vi "Process data - Overview v2.vi"() -> ()   [LabVIEW 2021]
uses:
  <vilib>/Utility/miscctls.llb/LV3DPointTypeDef.ctl
  <vilib>/Platform/TimedLoop/XDataNode/timing_clust.ctl
  <vilib>/Platform/TimedLoop/XDataNode/nitl_modes.ctl
  <vilib>/Platform/TimedLoop/XDataNode/wakeup.ctl
  <vilib>/picture/3D Picture Control/Object/Create Object (name).vi
  <vilib>/picture/3D Picture Control/Object/Create Object (drawable).vi
  <vilib>/picture/3D Picture Control/Object/Add Object (no reference).vi
  <vilib>/platform/TimedLoop/XDataNode/XDataNode.xnode
  <vilib>/Platform/TimedLoop/XDataNode/XDNodeRunTimeDep.lvlib
  <vilib>/picture/3D Picture Control/NI_3D Picture Control.lvlib
  <vilib>/gmath/NI_Gmath.lvlib
panel:
  out "IMU 2":refnum<vi>(3d-picture)
  in  "Enum 4":enum16{"None", "Disc", "Box", "STL"}(ring)=enum."Disc"
  out "X to N angle":dbl
  out "Magnetometer 2":refnum<vi>(3d-picture)
  in  "stop magnetometer":bool
  out "Magnetometer":refnum<vi>(3d-picture)
  out "Magnetometer corrected":refnum<vi>(3d-picture)
  in  "Calibrate":bool
  in  "Clear":bool
  in  "stop Accerelometer":bool
  in  "Enum 3":enum16{"None", "Disc", "Box", "STL"}(ring)=enum."Disc"
  out "FN RZRollY":dbl
  out "FN RYRollZ":dbl
  out "FN RXRollZ":dbl
  out "FN RZRollX":dbl
  out "FN RYRollX":dbl
  out "FN RXRollY":dbl
  in  "Camera Position":T1={"X"=1.0, "Y"=2.0, "Z"=5.0}
  out "FN ZRoll":dbl
  out "FN YRoll":dbl
  out "FN XRoll":dbl
  out "IMU":refnum<vi>(3d-picture)
  in  "DAQ Port":refnum<visa-resource-name>
  # "Other options"
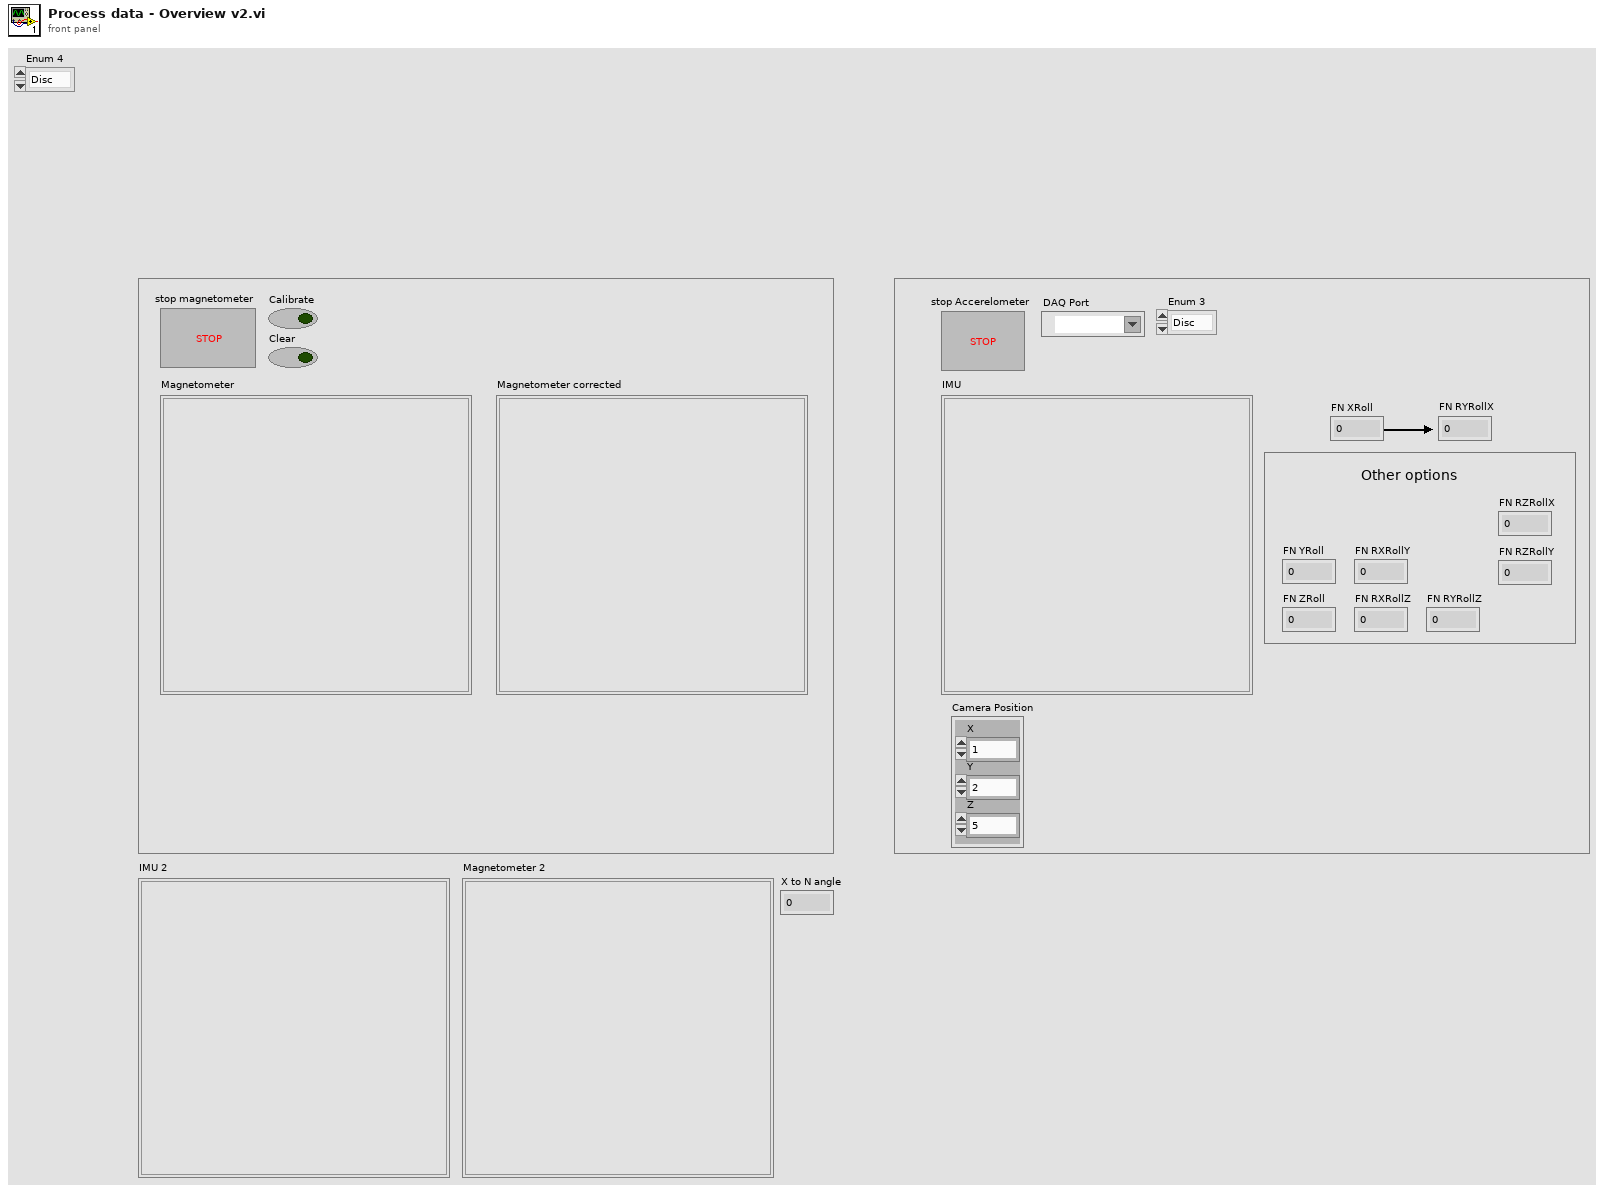
[diagram p1: front panel]
types:
  T1 = typedef "LV3DPointTypeDef.ctl" = cluster{"X":sgl, "Y":sgl, "Z":sgl}
  T2 = enum32{"Invalid", "Standard", "Closed", "Hidden", "Minimized", "Maximized"}
  T3 = cluster{"Red":sgl, "Green":sgl, "Blue":sgl, "Alpha":sgl}
  T4 = typedef "XDNodeRunTimeDep.lvlib/timing_clust.ctl" = cluster{"Expected End [f-1]":u64, "Actual End [f-1]":u64, "Finished Late? [f-1]":bool, "Expected End [i-1]":u64, "Actual End [i-1]":u64, "Finished Late? [i-1]":bool, "Expected Start [i]":u64, "Actual Start [i]":u64, "Expected Start [f]":u64, "Actual Start [f]":u64, "Source Name":string, "Structure Name":string, "Period":i64, "Deadline":i64, "Offset":i64, "Start":i64, "Priority":i32, "Timeout":i32, "Mode":T5, "Wakeup Reason":T6, "Error":errorcluster, "Source Type":string, "Secondary Source Type":string, "Global End Time":u64, "Global Start Time":u64, "Frame Duration":u64, "Iteration Duration":u64, "Assigned CPU":i32, "I/O Scan Engine Mode":u32}
  T5 = typedef "XDNodeRunTimeDep.lvlib/nitl_modes.ctl" = enum32{"No Change", "Process missed periods, maintain original phase", "Discard missed periods, maintain original phase", "Process missed periods, ignore original phase", "Discard missed periods, ignore original phase"}
  T6 = typedef "XDNodeRunTimeDep.lvlib/wakeup.ctl" = enum32{"Normal", "Aborted", "Asynchronous wakeup", "Timing source error", "Timed loop error", "Timeout"}
  T7 = cluster{"x0, y0, z0[0]":dbl, "x0, y0, z0[1]":dbl, "x0, y0, z0[2]":dbl}
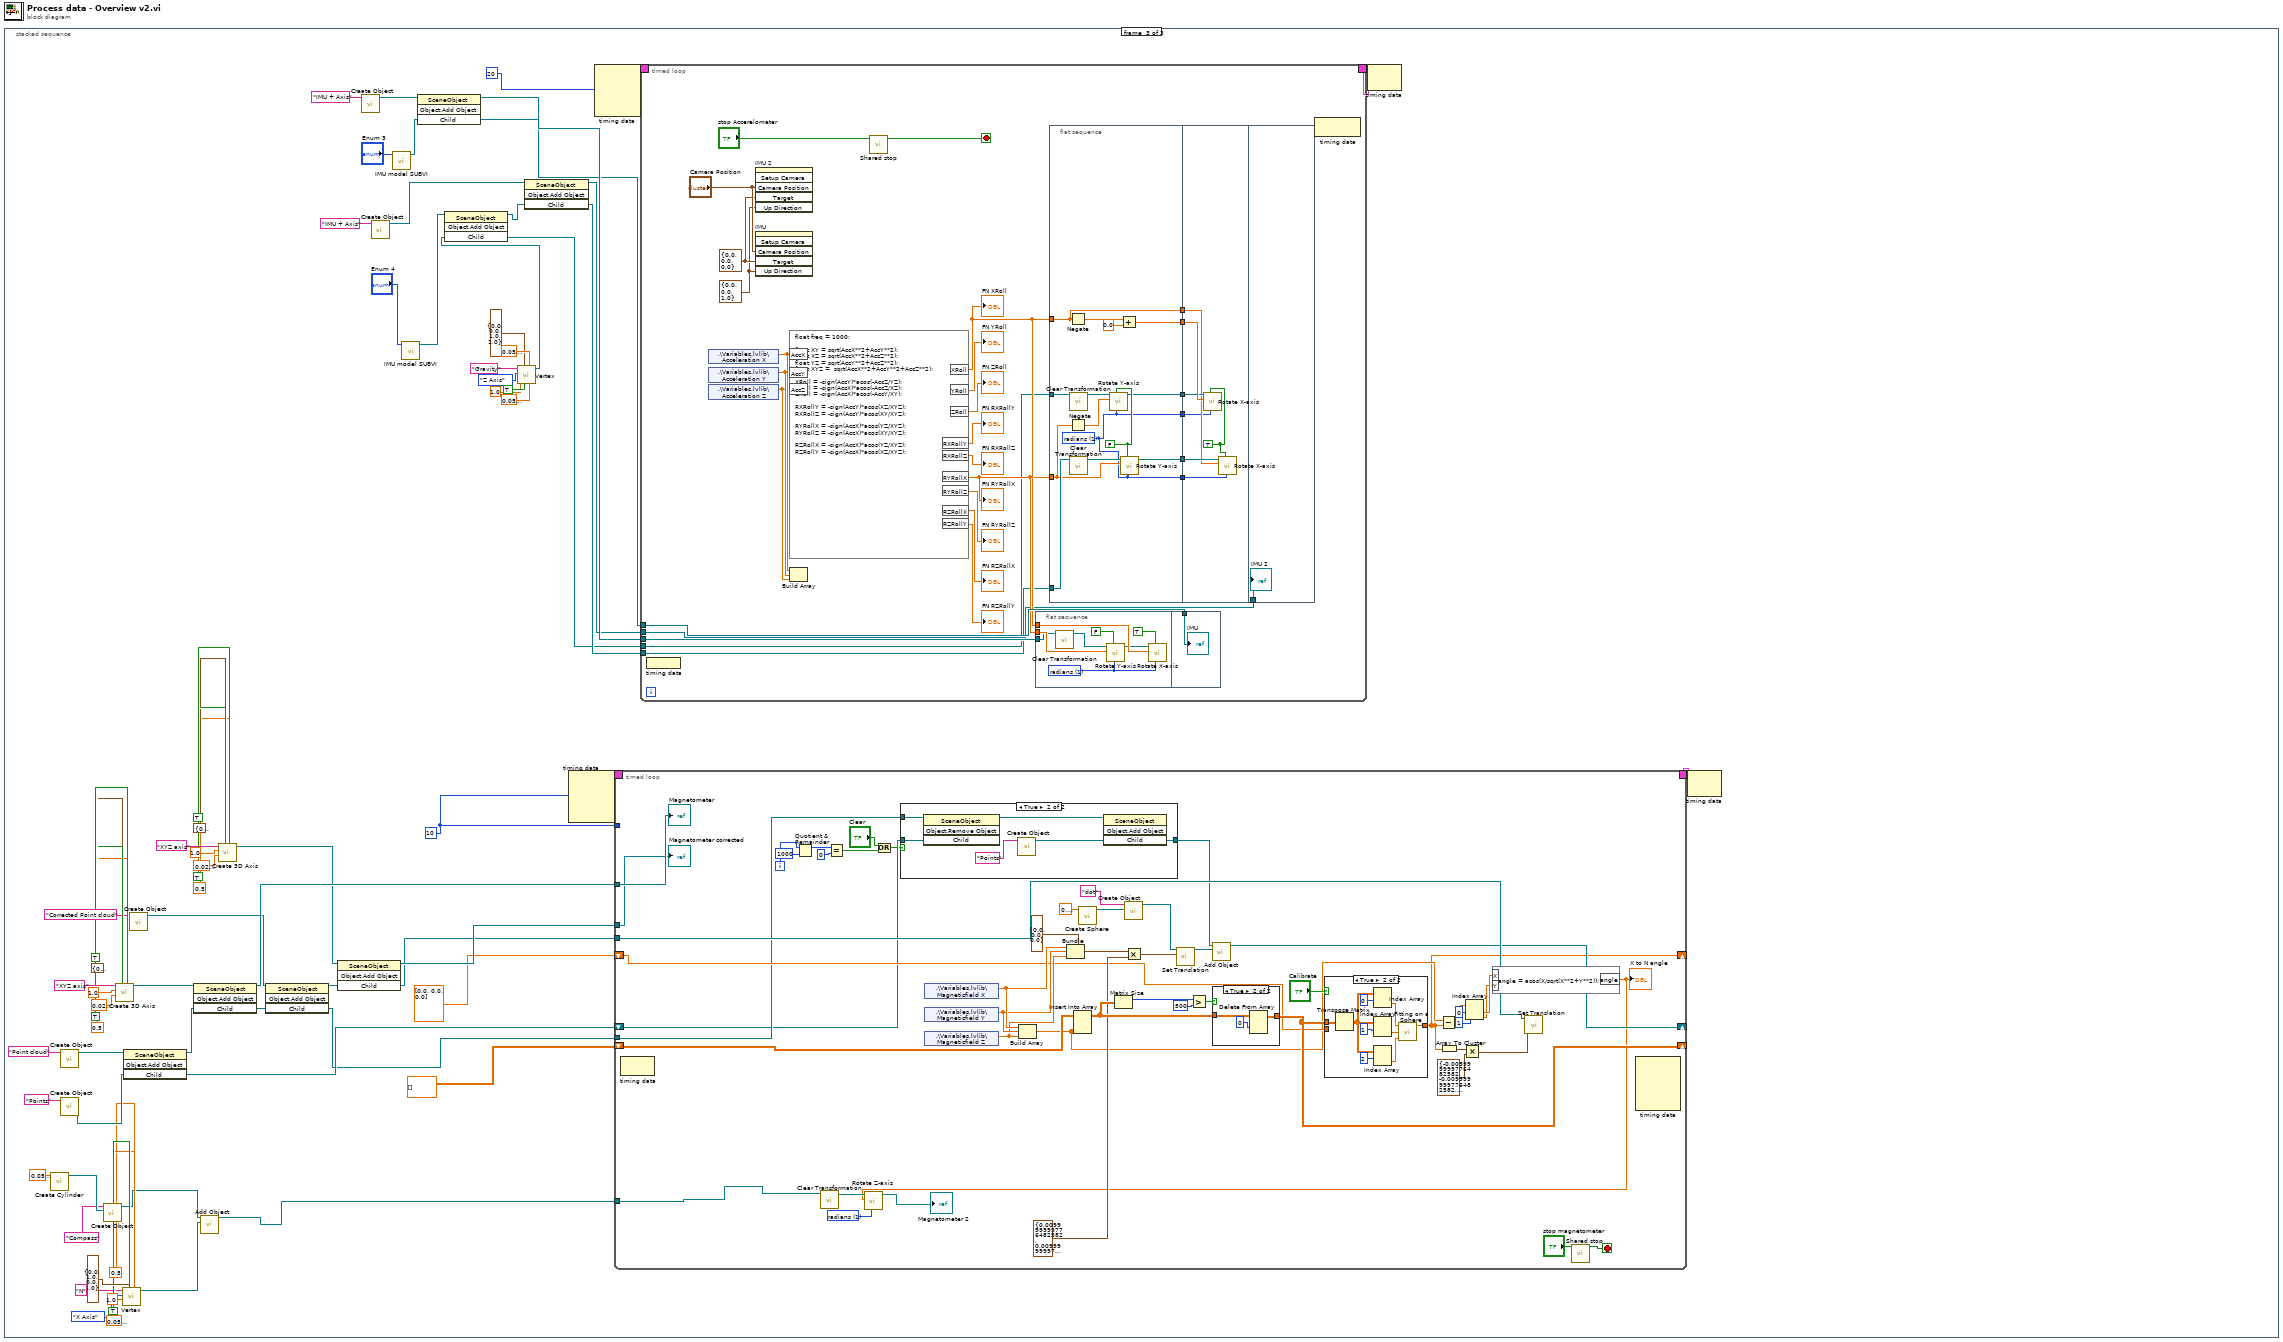
[diagram p0: block diagram]
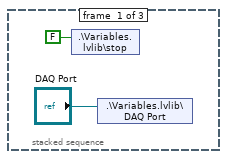
[diagram p2: hidden frame]
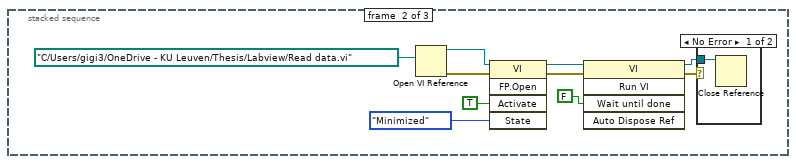
[diagram p3: hidden frame]
diagram:
  n1 = stacked-sequence {
    frame #0 {
      n2 = shared-variable ".\\Variables.lvlib\\stop"(FALSE ("stop")) -> ()  [unwired: 1 in, 1 out]
      n3 = shared-variable ".\\Variables.lvlib\\DAQ Port"("DAQ Port") -> ()  [unwired: 1 in, 1 out]
    }
    frame #1 {
      n4 = Open VI Reference(vi path=path "C:/Users/gigi3/OneDrive - KU Leuven/Thesis/Labview/Read data.vi") -> (vi reference=w12:refnum<vi>, error out=w4:errorcluster)  [unwired: 5 in]
      n5 = invoke class="VI" method="FP.Open"(reference=w12, error in=w4, "Activate"=TRUE ("Activate?"), "State"=T2."Minimized") -> (reference out=w11:refnum<vi>, error out=w5:errorcluster)  [unwired: 1 in, 3 out]
      n6 = invoke class="VI" method="Run VI"(reference=w11, error in=w5, "Wait until done"=FALSE ("Wait Until Done")) -> (reference out=w8:refnum<vi>, error out=w6:errorcluster)  [unwired: 2 in, 3 out]
      n7 = case shown="No Error" w6 {
        tunnel: w8 -> [w13 _]
        frame No Error {
          n8 = Close Reference(reference=w13) -> ()  [unwired: 1 in, 1 out]
        }
        frame Error {
        }
      }
    }
    frame #2 {
      w75 = i64 10 ("Period")
      n9 = call <vilib>:"Create Cylinder.vi"("Height"=sgl 0.05) -> ("New Cylinder Refnum"=w41:refnum<vi>)  [unwired: 9 in, 1 out]
      n10 = call-poly <vilib>:"Create Object.vi"("Name"="Point cloud") -> ("Scene:New Object"=w46:refnum<vi>)  [unwired: 9 in, 1 out]
      n11 = call-poly <vilib>:"Create Object.vi"("Name"="Points") -> ("Scene:New Object"=w48:refnum<vi>)  [unwired: 9 in, 1 out]
      n12 = call-poly <vilib>:"Create Object.vi"("Geometry"=w41, "Name"="Compass") -> ("Scene:New Object"=w32:refnum<vi>)  [unwired: 8 in, 1 out]
      n13 = call <vilib>:"Create 3D Axis.vi"("Character Size"=sgl 0.5, "Half plane?"=TRUE, "Axis label?"=TRUE, "Color"=T3 {"Red"=0.0, "Green"=1.0, "Blue"=0.0, "Alpha"=1.0}, "Radius"=sgl 0.03, "Length"=sgl 1.0, "Name"="XYZ axis") -> ("New Object Refnum"=w59:refnum<vi>)  [unwired: 3 in, 1 out]
      n14 = call "Vertex.vi"("Radius"=sgl 0.05, "Font Size"=sgl 0.5, "Vertex label?"=TRUE, "Color"=T3 {"Red"=0.0, "Green"=1.0, "Blue"=0.0, "Alpha"=1.0}, "Length"=sgl 1.0, "Enum"=enum16{"X Axis", "Y Axis", "Z Axis"}."X Axis", "Name"="N") -> ("New Object Refnum"=w31:refnum<vi>)  [unwired: 3 in, 1 out]
      n15 = invoke class="SceneObject" method="Object.Add Object"(reference=w46, "Child"=w48) -> (reference out=w47:refnum<vi>, "Child"=w45:refnum<vi>)  [unwired: 2 in, 2 out]
      n16 = call-poly <vilib>:"Create Object.vi"("Name"="Corrected Point cloud") -> ("Scene:New Object"=w55:refnum<vi>)  [unwired: 9 in, 1 out]
      n17 = invoke class="SceneObject" method="Object.Add Object"(reference=w59, "Child"=w47) -> (reference out=w58:refnum<vi>, "Child"=w50:refnum<vi>)  [unwired: 2 in, 2 out]
      n18 = call-poly <vilib>:"Add Object.vi"("New Object In"=w31, "Scene Object In"=w32) -> ("Scene Object Out"=w30:refnum<vi>)  [unwired: 8 in, 1 out]
      n19 = call <vilib>:"Create 3D Axis.vi"("Character Size"=sgl 0.5, "Half plane?"=TRUE, "Axis label?"=TRUE, "Color"=T3 {"Red"=0.0, "Green"=1.0, "Blue"=0.0, "Alpha"=1.0}, "Radius"=sgl 0.03, "Length"=sgl 1.0, "Name"="XYZ axis") -> ("New Object Refnum"=w54:refnum<vi>)  [unwired: 3 in, 1 out]
      n20 = invoke class="SceneObject" method="Object.Add Object"(reference=w55, "Child"=w50) -> (reference out=w53:refnum<vi>, "Child"=w44:refnum<vi>)  [unwired: 2 in, 2 out]
      n21 = invoke class="SceneObject" method="Object.Add Object"(reference=w54, "Child"=w53) -> (reference out=w52:refnum<vi>, "Child"=w51:refnum<vi>)  [unwired: 2 in, 2 out]
      n22 = call-poly <vilib>:"Create Object.vi"("Name"="IMU + Axis") -> ("Scene:New Object"=w78:refnum<vi>)  [unwired: 9 in, 1 out]
      n23 = call-poly <vilib>:"Create Object.vi"("Name"="IMU + Axis") -> ("Scene:New Object"=w23:refnum<vi>)  [unwired: 9 in, 1 out]
      n24 = call "IMU model SUBVI.vi"("Enum 3"="Enum 3") -> ("SceneObject out"=w79:refnum<vi>)  [unwired: 10 in]
      n25 = call "IMU model SUBVI.vi"("Enum 3"="Enum 4") -> ("SceneObject out"=w25:refnum<vi>)  [unwired: 10 in]
      n26 = invoke class="SceneObject" method="Object.Add Object"(reference=w78, "Child"=w79) -> (reference out=w80:refnum<vi>, "Child"=w81:refnum<vi>)  [unwired: 2 in, 2 out]
      n27 = call "Vertex.vi"("Radius"=sgl 0.05, "Font Size"=sgl 0.05, "Vertex label?"=TRUE, "Color"=T3 {"Red"=0.0, "Green"=0.0, "Blue"=1.0, "Alpha"=1.0}, "Length"=sgl 1.0, "Enum"=enum16{"X Axis", "Y Axis", "Z Axis"}."Z Axis", "Name"="Gravity") -> ("New Object Refnum"=w26:refnum<vi>)  [unwired: 3 in, 1 out]
      n28 = invoke class="SceneObject" method="Object.Add Object"(reference=w25, "Child"=w26) -> (reference out=w24:refnum<vi>, "Child"=w20:refnum<vi>)  [unwired: 2 in, 2 out]
      n29 = invoke class="SceneObject" method="Object.Add Object"(reference=w23, "Child"=w24) -> (reference out=w22:refnum<vi>, "Child"=w21:refnum<vi>)  [unwired: 2 in, 2 out]
      n30 = node-c288(w75) -> (w77:T4)  [unwired: 3 in]
      n31 = node-c288(i64 20 ("Period")) -> (w86:T4)  [unwired: 3 in]
      n32 = timed-loop {
        timing: w77 -> [_]
        timing-out: [_] -> w76
        tunnel: w75 -> [_]
        shift-right: [w131] -> _
        shift-left: dbl[][] [] -> [w136]
        tunnel: w58 -> [w118]
        tunnel: w52 -> [w117]
        tunnel: w51 -> [w116]
        shift-right: [w97] -> _
        shift-left: dbl[] [0.0, 0.0, 0.0] ("x0, y0, z0") -> [w114]
        tunnel: w44 -> [w112]
        shift-right: [w110] -> _
        shift-left: w45 -> [w109]
        tunnel: w30 -> [w91]
        i -> [w106]
        stop <- w102 stop-if-true
        w87 = u16 1 items=["degree", "radians"] ("angle unit")
        n33 = node-c288() -> ()  [unwired: 1 in, 1 out]
        n34 = Quotient & Remainder(x=w106, y=1000) -> (x-y*floor(x/y)=w103:i32)  [unwired: 1 out]
        n35 = call <vilib>:"Clear Transformation.vi"("Object Refnum In"=w91) -> ("Object Refnum Out"=w89:refnum<vi>)  [unwired: 9 in, 1 out]
        n36 = Equal?(x=w103, y=0) -> (x = y?=w105:bool)
        n37 = Or(x="Clear", y=w105) -> (x .or. y?=w108:bool)
        n38 = case shown="True" w108 {
          tunnel: w112 -> [_ w144]
          tunnel: [w138 w139] -> w111
          tunnel: w109 -> [w138 w140]
          frame False {
          }
          frame True {
            n39 = invoke class="SceneObject" method="Object.Remove Object"(reference=w144, "Child"=w140) -> (reference out=w142:refnum<vi>)  [unwired: 2 in, 3 out]
            n40 = call-poly <vilib>:"Create Object.vi"("Name"="Points") -> ("Scene:New Object"=w141:refnum<vi>)  [unwired: 9 in, 1 out]
            n41 = invoke class="SceneObject" method="Object.Add Object"(reference=w142, "Child"=w141) -> ("Child"=w139:refnum<vi>)  [unwired: 2 in, 3 out]
          }
        }
        n42 = shared-variable ".\\Variables.lvlib\\Magneticfield X"() -> (w122:dbl)  [unwired: 1 in, 1 out]
        n43 = shared-variable ".\\Variables.lvlib\\Magneticfield Y"() -> (w121:dbl)  [unwired: 1 in, 1 out]
        n44 = shared-variable ".\\Variables.lvlib\\Magneticfield Z"() -> (w120:dbl)  [unwired: 1 in, 1 out]
        n45 = Build Array(w122, w121, w120) -> (w101:dbl[])
        n46 = Bundle(cluster=cluster{"X":sgl, "Y":sgl, "Z":sgl} {"X"=0.0, "Y"=0.0, "Z"=0.0} ("Translation"), "X"=w122, "Y"=w121, "Z"=w120) -> (w125:cluster{"X":sgl, "Y":sgl, "Z":sgl})
        n47 = Insert Into Array(array=w136, new element=w101) -> (w135:dbl[][])  [unwired: 2 in]
        n48 = call <vilib>:"Create Sphere.vi"("Radius"=sgl 0.1) -> ("New Sphere Refnum"=w129:refnum<vi>)  [unwired: 9 in, 1 out]
        n49 = Matrix Size(0:w135) -> (1:w134:i32)  [unwired: 1 out]
        n50 = call-poly <vilib>:"Create Object.vi"("Geometry"=w129, "Name"="dot") -> ("Scene:New Object"=w127:refnum<vi>)  [unwired: 8 in, 1 out]
        n51 = Multiply(x=w125, y=cluster{"X":sgl, "Y":sgl, "Z":sgl} {"X"=0.01, "Y"=0.01, "Z"=0.01}) -> (x*y=w123:cluster{"X":sgl, "Y":sgl, "Z":sgl})
        n52 = call <vilib>:"Set Translation.vi"("Translation"=w123, "Scene Object"=w127) -> ("Translated Object"=w126:refnum<vi>)  [unwired: 8 in, 1 out]
        n53 = Greater?(x=w134, y=500) -> (0:w132:bool)
        n54 = call-poly <vilib>:"Add Object.vi"("New Object In"=w126, "Scene Object In"=w111) -> ("Scene Object Out"=w110:refnum<vi>)  [unwired: 8 in, 1 out]
        n55 = case shown="True" w132 {
          tunnel: w135 -> [w155 w158]
          tunnel: [w155 w156] -> w131
          frame False {
          }
          frame True {
            n56 = Delete From Array(array=w158, index (row)=0) -> (array with subset deleted=w156:dbl[][])  [unwired: 2 in, 1 out]
          }
        }
        n57 = case shown="True" "Calibrate" {
          tunnel: w131 -> [_ w154]
          tunnel: w114 -> [w145 _]
          tunnel: [w145 w146] -> w97
          frame False {
          }
          frame True {
            n58 = Transpose Matrix(1:w154) -> (0:w149:dbl[][])
            n59 = Index Array(array=w149, index (row)=0) -> (element=w153:dbl[])  [unwired: 1 in]
            n60 = Index Array(array=w149, index (row)=1) -> (element=w148:dbl[])  [unwired: 1 in]
            n61 = Index Array(array=w149, index (row)=2) -> (element=w147:dbl[])  [unwired: 1 in]
            n62 = call <vilib>:"Fitting on a Sphere.vi"("Z"=w147, "Y"=w148, "X"=w153) -> ("x0, y0, z0"=w146:dbl[])  [unwired: 2 out]
          }
        }
        n63 = Subtract(x=w101, y=w97) -> (x-y=w96:dbl[])
        n64 = Array To Cluster(array=w97) -> (cluster=w99:T7)
        n65 = Multiply(x=w99, y=cluster{"X":sgl, "Y":sgl, "Z":sgl} {"X"=-0.01, "Y"=-0.01, "Z"=-0.01}) -> (x*y=w98:cluster{dbl, dbl, dbl})
        n66 = Index Array(array=w96, index #1=0 ("index"), index #2=1 ("index")) -> (element #1=w93:dbl, element #2=w92:dbl)
        n67 = formula code="angle = acos(X/sqrt(X**2+Y**2));"("X"=w93, "Y"=w92) -> ("angle"=w88:dbl)
        "X to N angle" <- w88
        n68 = call <vilib>:"Rotate Z-axis.vi"("angle unit"=w87, "angle"=w88, "Scene Object In"=w89) -> ("Scene Object Out"=→"Magnetometer 2":refnum<vi>)  [unwired: 7 in, 1 out]
        n69 = call <vilib>:"Set Translation.vi"("Translation"=w98, "Scene Object"=w116) -> ()  [unwired: 8 in, 2 out]
        n70 = call "Shared stop.vi"("stop"="stop magnetometer") -> ("stop 2"=w102:bool)  [unwired: 10 in]
        n71 = node-c288() -> ()  [unwired: 5 in, 1 out]
        "Magnetometer" <- w118
        "Magnetometer corrected" <- w117
      }
      n72 = timed-loop {
        timing: w86 -> [_]
        timing-out: [_] -> w85
        tunnel: w80 -> [w184]
        tunnel: w81 -> [w185]
        tunnel: w22 -> [w179]
        tunnel: w21 -> [w178]
        tunnel: w20 -> [w171]
        stop <- w182 stop-if-true
        w172 = T1 {"X"=0.0, "Y"=0.0, "Z"=1.0} ("Up Direction")
        w173 = T1 {"X"=0.0, "Y"=0.0, "Z"=0.0} ("Target")
        n73 = node-c288() -> ()  [unwired: 1 in]
        n74 = shared-variable ".\\Variables.lvlib\\Acceleration X"() -> (w177:dbl)  [unwired: 1 in, 1 out]
        n75 = shared-variable ".\\Variables.lvlib\\Acceleration Y"() -> (w176:dbl)  [unwired: 1 in, 1 out]
        n76 = shared-variable ".\\Variables.lvlib\\Acceleration Z"() -> (w175:dbl)  [unwired: 1 in, 1 out]
        n77 = invoke on="IMU 2" class="SceneGraphDisp (strict)" method="Setup Camera"("Camera Position"="Camera Position", "Target"=w173, "Up Direction"=w172) -> ()  [unwired: 3 in, 6 out]
        n78 = invoke on="IMU" class="SceneGraphDisp (strict)" method="Setup Camera"("Camera Position"="Camera Position", "Target"=w173, "Up Direction"=w172) -> ()  [unwired: 3 in, 6 out]
        n79 = formula code="float freq = 1000;\n\nfloat XY = sqrt(AccX**2+AccY**2);\nfloat XZ = sqrt(AccX**2+AccZ**2);\nfloat YZ = sqrt(AccY**2+AccZ**2);\nfloat XYZ =  sqrt(AccX**2+AccY**2+AccZ**2);\n\nXRoll = -sign(AccY)*acos(-AccZ/YZ);\nYRoll = -sign(AccX)*acos(-AccZ/XZ);\nZRoll = -sign(AccX)*acos(-AccY/XY);\n\nRXRollY = -sign(AccY)*acos(XZ/XYZ);\nRXRollZ = -sign(AccY)*acos(XY/XYZ);\n\nRYRollX = -sign(AccX)*acos(YZ/XYZ);\nRYRollZ = -sign(AccX)*acos(XY/XYZ);\n\nRZRollX = -sign(AccX)*acos(YZ/XYZ);\nRZRollY = -sign(AccX)*acos(XZ/XYZ);"("AccX"=w177, "AccY"=w176, "AccZ"=w175) -> ("XRoll"=w181:dbl, "YRoll"=→"FN YRoll":dbl, "ZRoll"=→"FN ZRoll":dbl, "RXRollY"=→"FN RXRollY":dbl, "RYRollX"=w180:dbl, "RZRollX"=→"FN RZRollX":dbl, "RXRollZ"=→"FN RXRollZ":dbl, "RYRollZ"=→"FN RYRollZ":dbl, "RZRollY"=→"FN RZRollY":dbl)
        "FN XRoll" <- w181
        "FN RYRollX" <- w180
        n80 = Build Array(w177, w176, w175) -> ()  [unwired: 1 out]
        n81 = call "Shared stop.vi"("stop"="stop Accerelometer") -> ("stop 2"=w182:bool)  [unwired: 10 in]
        n82 = flat-sequence {
          tunnel: w181 -> [w222]
          tunnel: w180 -> [w220]
          tunnel: w185 -> [w217]
          tunnel: w184 -> [w223]
          frame #0 {
            w219 = u16 1 items=["degree", "radians"] ("angle unit")
            n83 = call <vilib>:"Clear Transformation.vi"("Object Refnum In"=w217) -> ("Object Refnum Out"=w216:refnum<vi>)  [unwired: 9 in, 1 out]
            n84 = call <vilib>:"Rotate Y-axis.vi"("angle unit"=w219, "Relative?"=FALSE, "angle"=w220, "Scene Object In"=w216) -> ("Scene Object Out"=w215:refnum<vi>)  [unwired: 6 in, 1 out]
            n85 = call <vilib>:"Rotate X-axis.vi"("angle unit"=w219, "Relative?"=TRUE, "angle"=w222, "Scene Object In"=w215) -> ()  [unwired: 6 in, 2 out]
          }
          frame #1 {
            "IMU" <- w223
          }
        }
        n86 = flat-sequence {
          tunnel: w178 -> [w206]
          tunnel: w181 -> [w195]
          tunnel: w180 -> [w202]
          tunnel: w171 -> [w200]
          tunnel: [w198] -> w170
          tunnel: [w197] -> w169
          tunnel: [w196] -> w168
          tunnel: [w195] -> w167
          tunnel: [w194] -> w166
          tunnel: [w194] -> w165
          tunnel: w170 -> [w213]
          tunnel: w169 -> [w212]
          tunnel: w168 -> [w211]
          tunnel: w167 -> [w210]
          tunnel: w166 -> [w209]
          tunnel: w165 -> [w208]
          tunnel: w179 -> [w214]
          frame #0 {
            w199 = FALSE ("Relative?")
            w194 = u16 1 items=["degree", "radians"] ("angle unit")
            n87 = Negate(x=w195) -> (-x=w204:dbl)
            n88 = Negate(x=w202) -> (-x=w203:dbl)
            n89 = call <vilib>:"Clear Transformation.vi"("Object Refnum In"=w200) -> ("Object Refnum Out"=w201:refnum<vi>)  [unwired: 9 in, 1 out]
            n90 = call <vilib>:"Clear Transformation.vi"("Object Refnum In"=w206) -> ("Object Refnum Out"=w205:refnum<vi>)  [unwired: 9 in, 1 out]
            n91 = call <vilib>:"Rotate Y-axis.vi"("angle unit"=w194, "Relative?"=w199, "angle"=w203, "Scene Object In"=w201) -> ("Scene Object Out"=w197:refnum<vi>)  [unwired: 6 in, 1 out]
            n92 = Add(x=w204, y=0.0) -> (x+y=w198:dbl)
            n93 = call <vilib>:"Rotate Y-axis.vi"("angle unit"=w194, "Relative?"=w199, "angle"=w202, "Scene Object In"=w205) -> ("Scene Object Out"=w196:refnum<vi>)  [unwired: 6 in, 1 out]
          }
          frame #1 {
            w207 = TRUE ("Relative?")
            n94 = call <vilib>:"Rotate X-axis.vi"("angle unit"=w208, "Relative?"=w207, "angle"=w213, "Scene Object In"=w212) -> ()  [unwired: 6 in, 2 out]
            n95 = call <vilib>:"Rotate X-axis.vi"("angle unit"=w209, "Relative?"=w207, "angle"=w210, "Scene Object In"=w211) -> ()  [unwired: 6 in, 2 out]
          }
          frame #2 {
            "IMU 2" <- w214
          }
        }
        n96 = node-c288() -> ()  [unwired: 1 in, 1 out]
      }
      n97 = node-c288(w85) -> ()  [unwired: 1 out]
      n98 = node-c288(w76) -> ()  [unwired: 1 out]
    }
  }
